vi "write_params.vi"(8 "error in (no error)":errorcluster, 10 "params":T1={"alpha"=1.0, "fit_intercept"=TRUE, "max_iter"=100.0, "tol"=0.0001, "warm_start"=FALSE, "verbose"=0.0}, 11 "PoissonRegressor in":refnum<class "PoissonRegressor.lvclass">) -> (0 "error out":errorcluster, 3 "PoissonRegressor out":refnum<class "PoissonRegressor.lvclass">)   [LabVIEW 2020, in "PoissonRegressor.lvclass"]
uses:
  PoissonRegressor.lvclass
  Controls/poisson_regressor_params.ctl
  PoissonRegressor.lvclass/PoissonRegressor.ctl
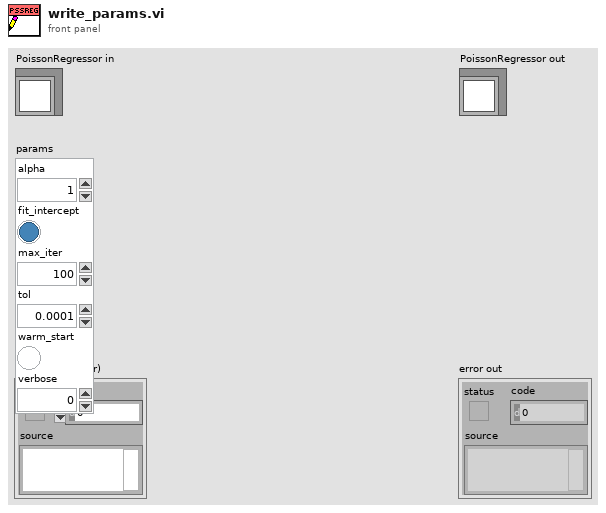
[diagram p1: front panel]
types:
  T1 = typedef "poisson_regressor_params.ctl" = cluster{"alpha":dbl, "fit_intercept":bool, "max_iter":dbl, "tol":dbl, "warm_start":bool, "verbose":dbl}
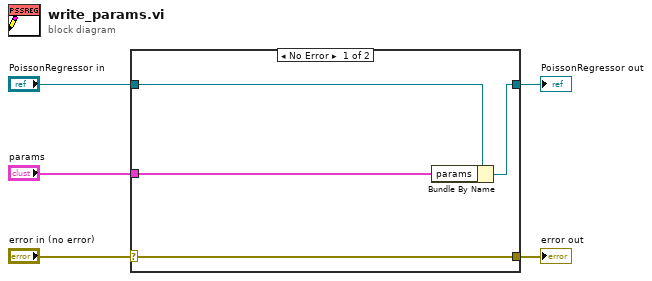
[diagram p0: block diagram]
diagram:
  n1 = case shown="No Error" "error in (no error)" {
    selector: "error in (no error)" -> [w9 w10]
    tunnel: [w9 w10] -> w4
    tunnel: [w7 w11] -> w2
    tunnel: "PoissonRegressor in" -> [w8 w11]
    tunnel: "params" -> [w6 _]
    frame No Error {
      n2 = Bundle By Name(cluster=w8, "params"=w6) -> (w7:refnum<class "PoissonRegressor.lvclass">)
    }
    frame Error {
    }
  }
  "error out" <- w4
  "PoissonRegressor out" <- w2
